vi "MakeButtonTransitions.vi"(9 "Simplified":bool, 11 "NavigationItem":T1) -> (3 "PlantUML":string)   [LabVIEW 2021, in "ButtonBarFlow.lvlib"]
uses:
  ButtonBarFlow.lvlib
  TAFAOModule_GUI_VerticalButtonBar/VerticalButtonBar/ButtonCollection/ButtonDefinition.ctl
  TAFAOModule_GUI_VerticalButtonBar/VerticalButtonBar/ButtonCollection/ButtonCollection.lvclass
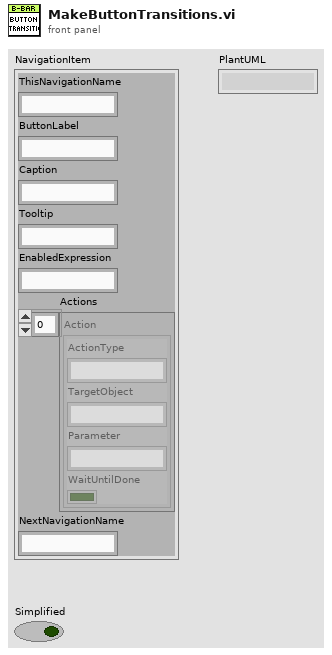
[diagram p1: front panel]
types:
  T1 = typedef "ButtonCollection.lvclass/ButtonDefinition.ctl" = cluster{"ThisNavigationName":string, "ButtonLabel":string, "Caption":string, "Tooltip":string, "EnabledExpression":string, "Actions":cluster{"ActionType":string, "TargetObject":string, "Parameter":string, "WaitUntilDone":bool}[], "NextNavigationName":string}
  T2 = cluster{"ActionType":string, "TargetObject":string, "Parameter":string, "WaitUntilDone":bool}[]
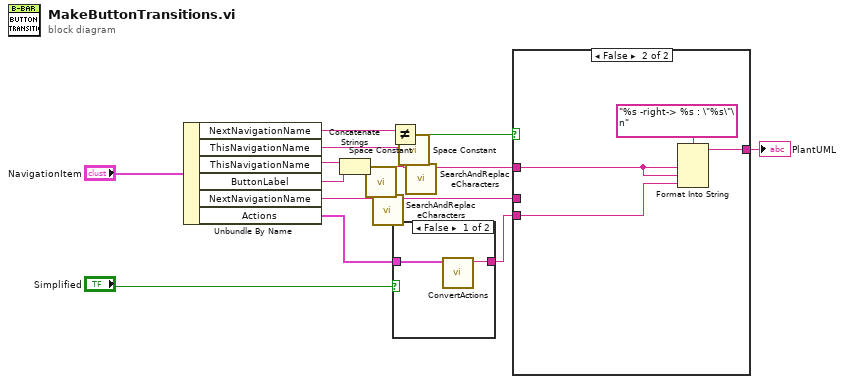
[diagram p0: block diagram]
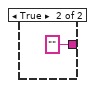
[diagram p2: hidden frame]
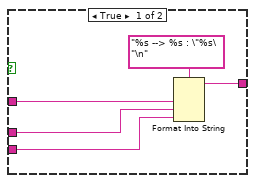
[diagram p3: hidden frame]
diagram:
  n1 = Unbundle By Name("NavigationItem") -> ("NextNavigationName"=w12:string, "ThisNavigationName"=w13:string, "ThisNavigationName"=w16:string, "ButtonLabel"=w10:string, "NextNavigationName"=w3:string, "Actions"=w15:T2)
  n2 = Concatenate Strings(w16, w10) -> (w8:string)
  n3 = call <vilib>:"Space Constant.vi"() -> ("String"=w6:string)
  n4 = call "SearchAndReplaceCharacters.vi"("CharactersToSearch"=w6, "StringIn"=w3) -> ("ResultString"=w5:string)  [unwired: 9 in]
  n5 = Not Equal?(x=w12, y=w13) -> (x != y?=w11:bool)
  n6 = case shown="False" "Simplified" {
    tunnel: w15 -> [w18 _]
    tunnel: [w17 "" ("ActionString")] -> w14
    frame False {
      n7 = call "ConvertActions.vi"("Actions"=w18) -> ("ActionString"=w17:string)  [unwired: 10 in]
    }
    frame True {
    }
  }
  n8 = call <vilib>:"Space Constant.vi"() -> ("String"=w9:string)
  n9 = call "SearchAndReplaceCharacters.vi"("CharactersToSearch"=w9, "StringIn"=w8) -> ("ResultString"=w7:string)  [unwired: 9 in]
  n10 = case shown="False" w11 {
    tunnel: [w23 w27] -> w2
    tunnel: w7 -> [w22 w25]
    tunnel: w5 -> [w21 _]
    tunnel: w14 -> [w20 w26]
    frame True {
      n11 = Format Into String(format string="%s --> %s : \"%s\"\n", w22, w21, w20) -> (resulting string=w23:string)  [unwired: 2 in, 1 out]
    }
    frame False {
      n12 = Format Into String(format string="%s -right-> %s : \"%s\"\n", w25, w25, w26) -> (resulting string=w27:string)  [unwired: 2 in, 1 out]
    }
  }
  "PlantUML" <- w2
